vi "PlayAlarmSound.vi"(8 "Error In":errorcluster, 10 "Alarm Sound Delay (sec)":dbl, 11 "Alarm Sound File Path":path) -> (0 "Error Out":errorcluster)   [LabVIEW 2012]
uses:
  libs/LV-Utilities/LV-Utilities.lvlib
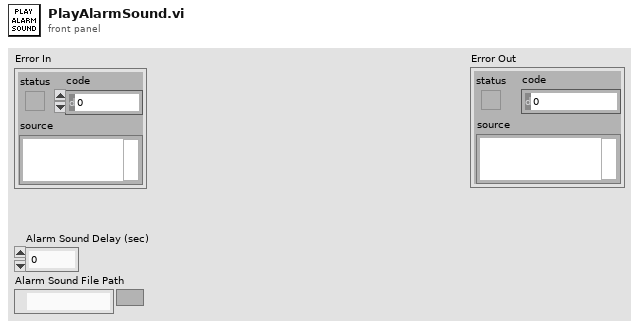
[diagram p1: front panel]
types:
  T1 = typedef "Sound Output Task ID.ctl" = u32
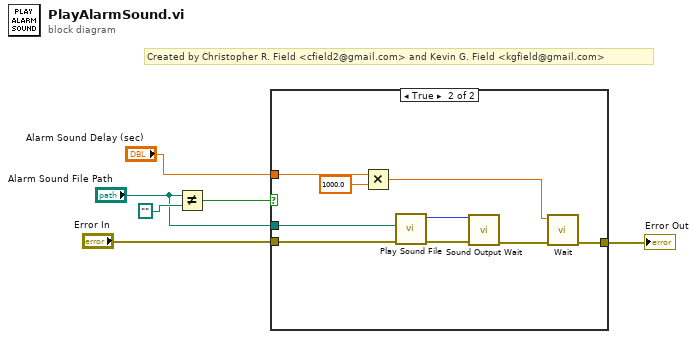
[diagram p0: block diagram]
diagram:
  # "Created by Christopher R. Field <cfield2@gmail.com> and Kevin G. Field <kgfield@gmail.com>"
  n1 = Not Equal?(x="Alarm Sound File Path", y=path "") -> (x != y?=w2:bool)
  n2 = case shown="True" w2 {
    tunnel: "Alarm Sound Delay (sec)" -> [_ w13]
    tunnel: "Error In" -> [w7 w10]
    tunnel: [w7 w9] -> w4
    tunnel: "Alarm Sound File Path" -> [_ w8]
    frame False {
    }
    frame True {
      n3 = Multiply(x=w13, y=1000.0) -> (x*y=w14:dbl)
      n4 = call <vilib>:"Play Sound File.vi"("error in (no error)"=w10, "path"=w8) -> ("error out"=w12:errorcluster, "task ID"=w16:T1)  [unwired: 8 in]
      n5 = call <vilib>:"Sound Output Wait.vi"("error in (no error)"=w12, "task ID"=w16) -> ("error out"=w11:errorcluster)  [unwired: 8 in, 1 out]
      n6 = call "Wait.vi"("Error In"=w11, "Wait Time (msec)"=w14) -> ("Error Out"=w9:errorcluster)  [unwired: 9 in]
    }
  }
  "Error Out" <- w4
